vi "pirometer 2.2_MAIN.vi"() -> ()   [LabVIEW 2013]
doc: "Пирометр 2.2, разработан в ЛФВЭ ОИЯИ 2013"
uses:
  pirometer typedef1.ctl
  <vilib>/Utility/error.llb/DialogType.ctl
  <vilib>/Instr/_visa.llb/VISA Configure Serial Port (Instr).vi
  <vilib>/ptbypt/NI_PtbyPt.lvlib
panel:
  in  "Гр2":bool=TRUE
  in  "Гр1":bool=TRUE
  out "Ошибка  прибора":bool
  in  "Недопустимая \nразница между\n показаниями":u8=35
  in  "Снимок экрана":bool
  in  "Мин\n  d/dt":dbl=-0.02 min=-200.0 max=200.0 step=0.01 format="%#.3g"
  in  "Макс\n  d/dt":dbl=0.02 min=-200.0 max=200.0 step=0.01 format="%#.3g"
  out "d/dt right scale":dbl(slide) min=-0.20900000000000002 max=0.196 scale=-0.02..0.02
  out "d/dt":dynamicdata(graph)
  out "gradusnik 2":dbl(slide) scale=-3.0..35.0
  in  "Мин. Т":i8=10
  in  "Stop":bool
  out "gradusnik":dbl(slide) scale=-3.0..35.0
  in  "Усреднение d/dt":u16=25
  in  "Усреднение T по":u8=50
  out "Средняя T":dbl format="%0.2f"
  in  "Макс.Т":i8=35
  out "Температура":dynamicdata(graph)
  in  "Запись в файл":bool
  out "сек.":string="20"
  out "мин.":string="3"
  out "часы":string
  in  "xScale +":bool
  in  "Добавить время":dbl(ring)=60.0 items=["1 сек."=1.0, "10 сек."=10.0, "1 мин."=60.0, "5 мин."=300.0, "10 мин."=600.0]
  in  "xScale -":bool
  out "Текущая T":dbl format="%0.2f"
  in  "Порт":refnum<visa-resource-name>="COM7"
  out "Соединение":bool
  out "Чтение":bool
  out "Расположение файла":path=path "Запись в файл не включена..."
  in  "Бод":u32=9600
  out "d/dt":dbl format="%#.3f"
  out "Exitting":string="Остановка программы..."
  in  "index of current arr element":i32
  out "i":i32
  in  "number of data sample":u64
  out "refnum out":refnum<file>
  in  "fl_1":bool
  out "Temper.":dbl
  out "Err msg":string=" INSTRUCTIONS:\r\rNormal Use:  When using subVIs that incorporate the error in/error out (or error I/O) structure, place this handler where you want to inform the user of an error, typically at the end of the I/O data path, as the last action of the program.  If the error in error? is ERROR, the handler creates a message describing the error and its source.  If the type of dialog = 1 (default), the message is displayed to the user, who can only acknowedge it.  If the type = 2, the user can acknowledge the message or abort execution; aborting a program with active I/O is not recommended.  If the type = 0, no message is displayed; this is used to process the error programmatically, and the error out cluster elements are wired to individual terminals for that reason.  \r\rOther Use:\n\r\nlocal testing.  To test the error code of a subVI or function that does not have the error I/O structure, you can wire its error code and a source string to the local error code and error source inputs.  If error in error? indicates no error and error code is not equal to 0, the local code and source are substituted for the error in values, and error? is set TRUE (ERROR)."
  # "°С"
  # "°С"
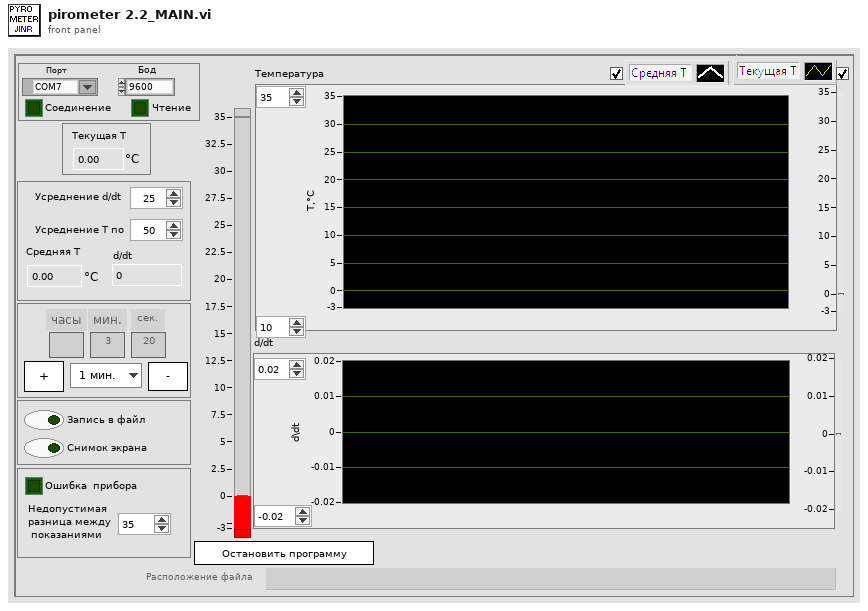
[diagram p1: front panel]
types:
  T1 = typedef "pirometer typedef1.ctl" = enum16{"Initialize", "Read port", "Averaging", "Create graph", "Save to file", "Stop", "ScreenCapture", "Err handle"}
  T2 = typedef "DialogType.ctl" = u16
  T3 = typedef "imagedata.ctl" = cluster{"image type":i32, "image depth":i32, "image":u8[], "mask":u8[], "colors":u32[], "Rectangle":cluster{"left":i16, "top":i16, "right":i16, "bottom":i16}}
  T4 = typedef "LVDateTimeRec.ctl" = cluster{"fractional second":dbl, "second":i32, "minute":i32, "hour":i32, "day of month":i32, "month":i32, "year":i32, "day of week":i32, "day of year":i32, "DST":i32}
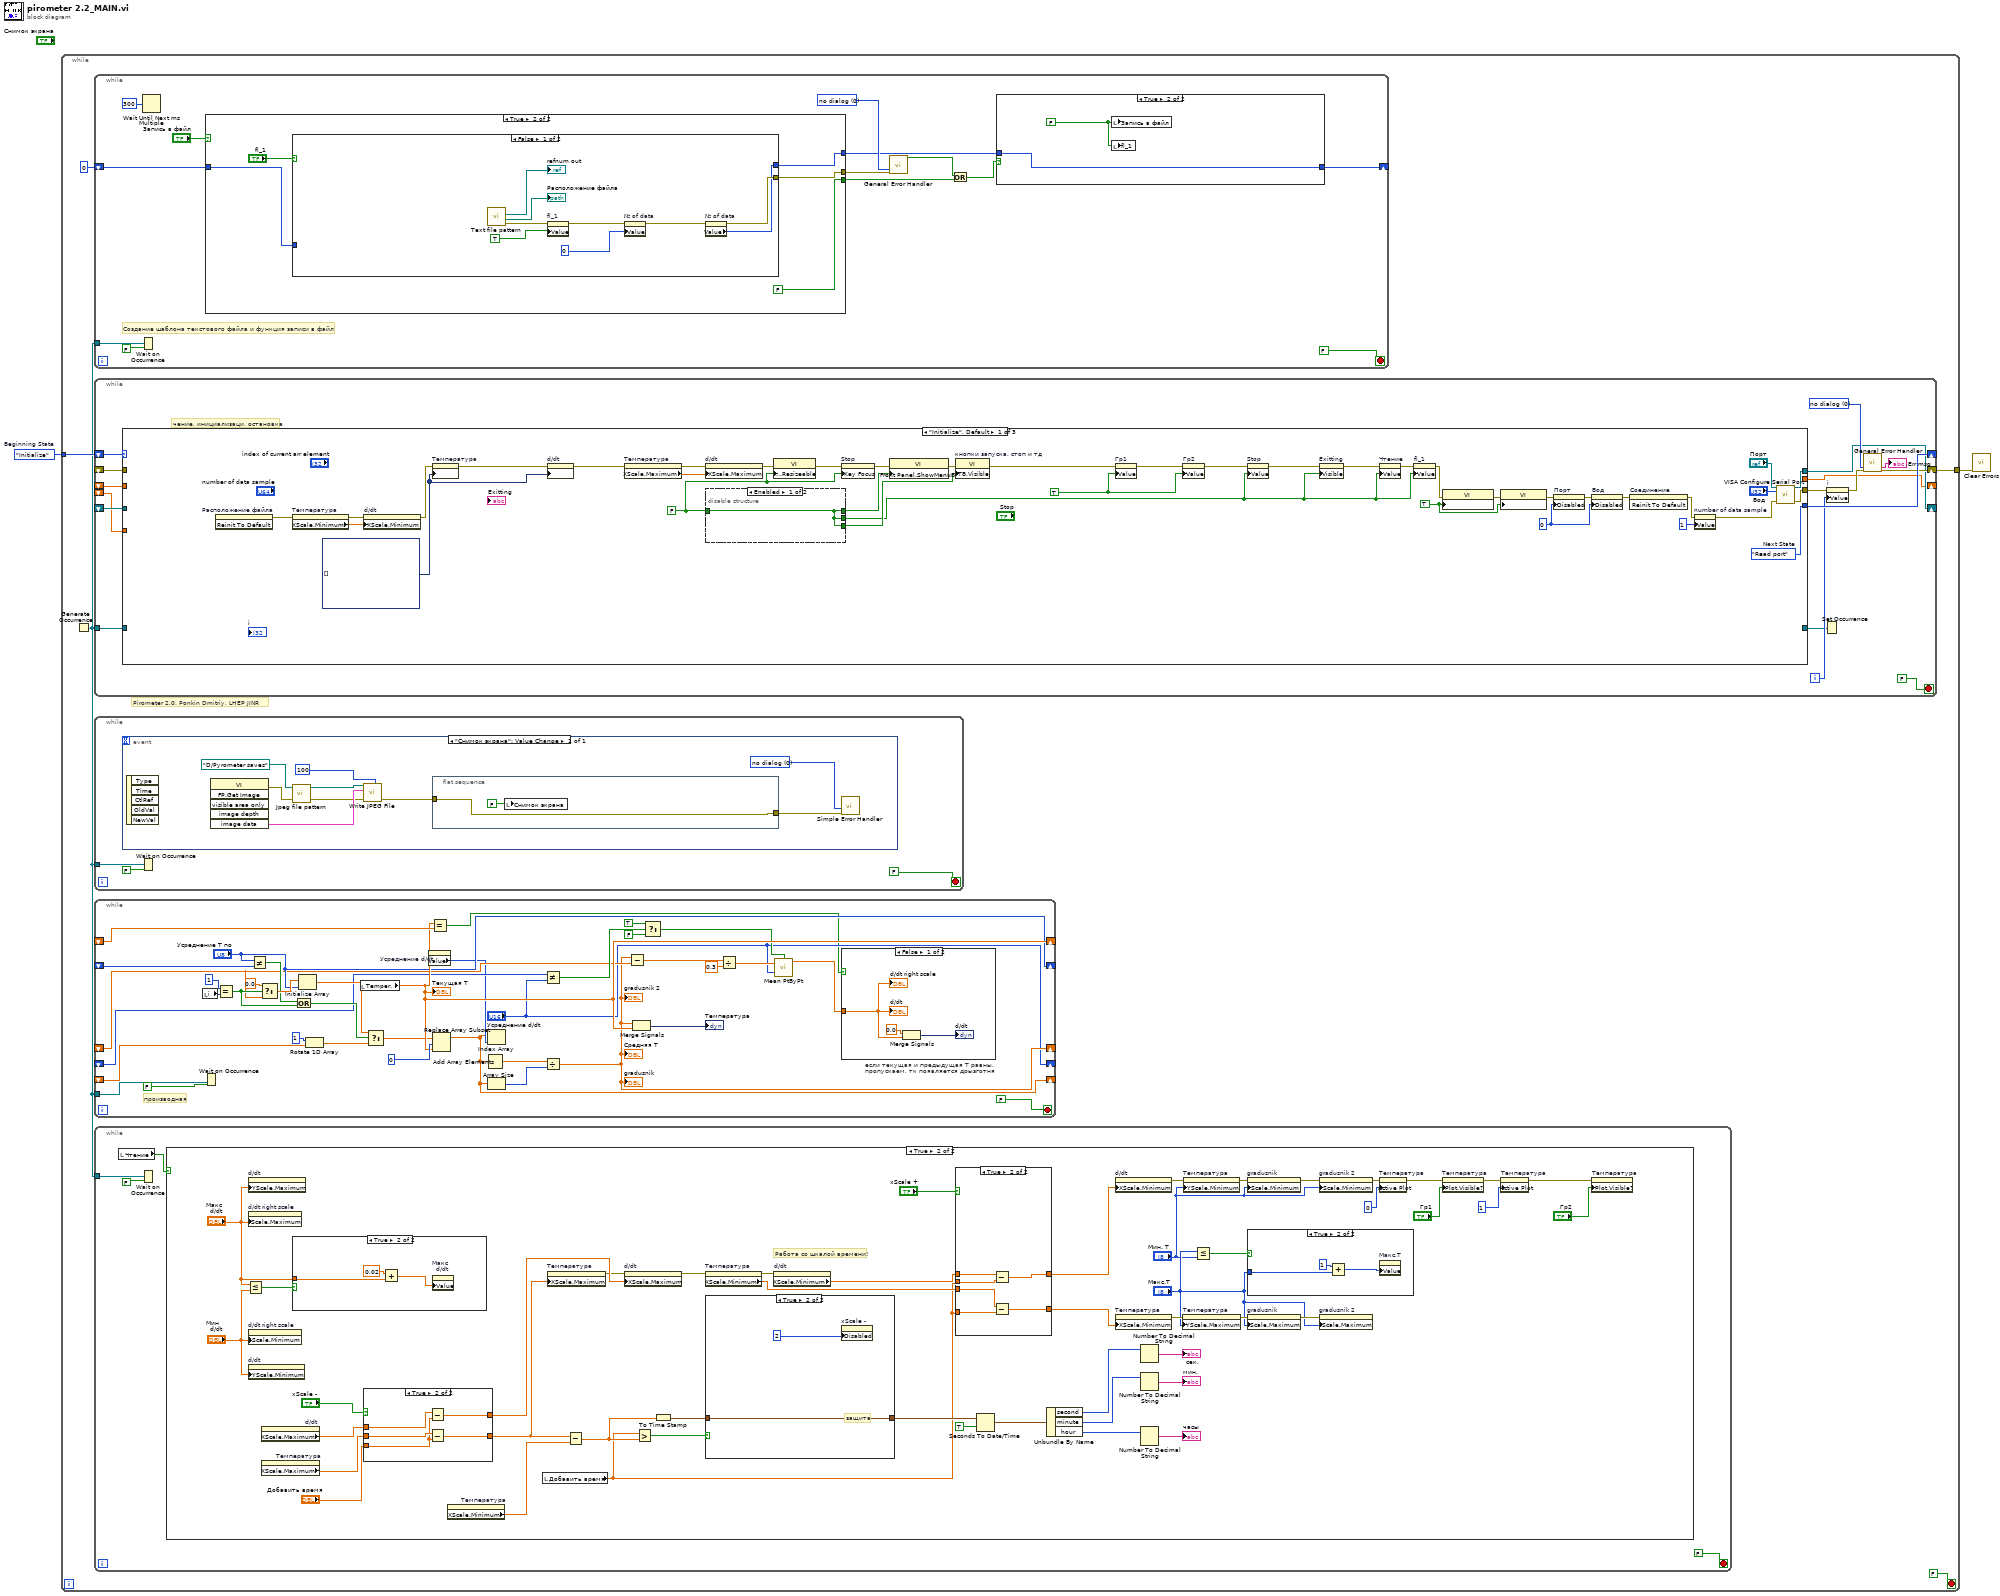
[diagram p0: block diagram]
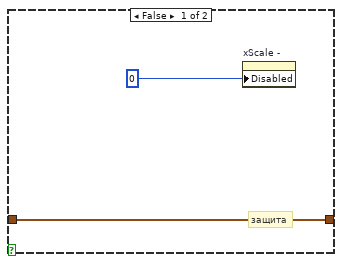
[diagram p6: hidden frame]
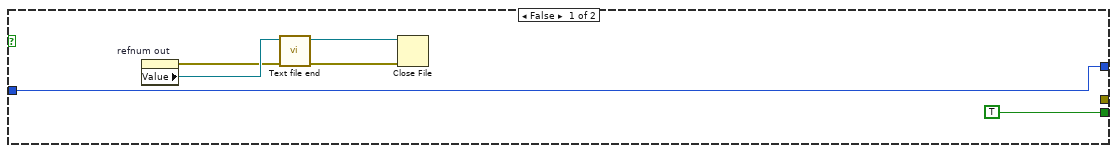
[diagram p10: hidden frame]
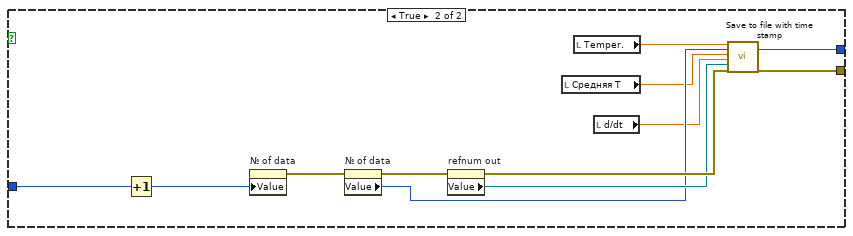
[diagram p11: hidden frame]
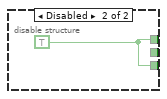
[diagram p12: hidden frame]
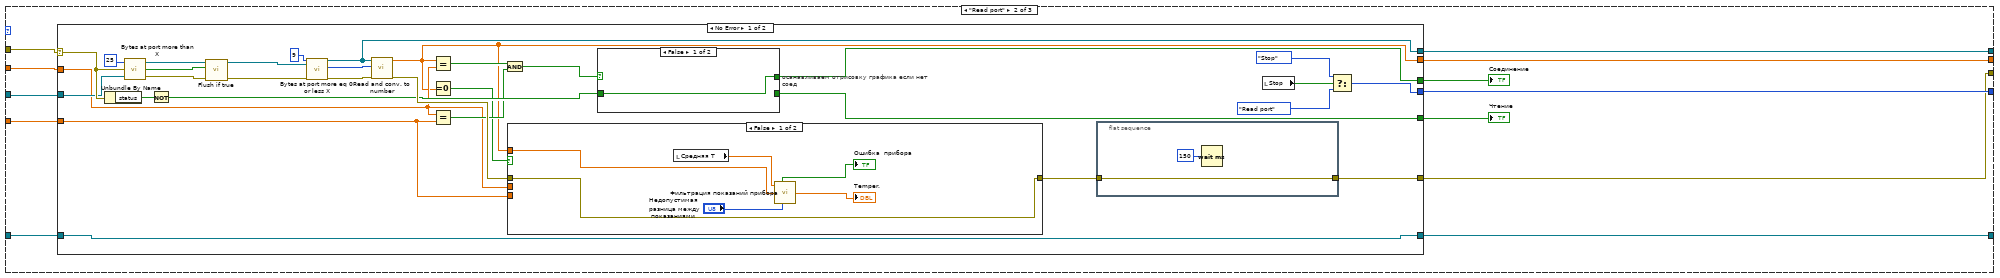
[diagram p13: hidden frame]
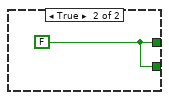
[diagram p14: hidden frame]
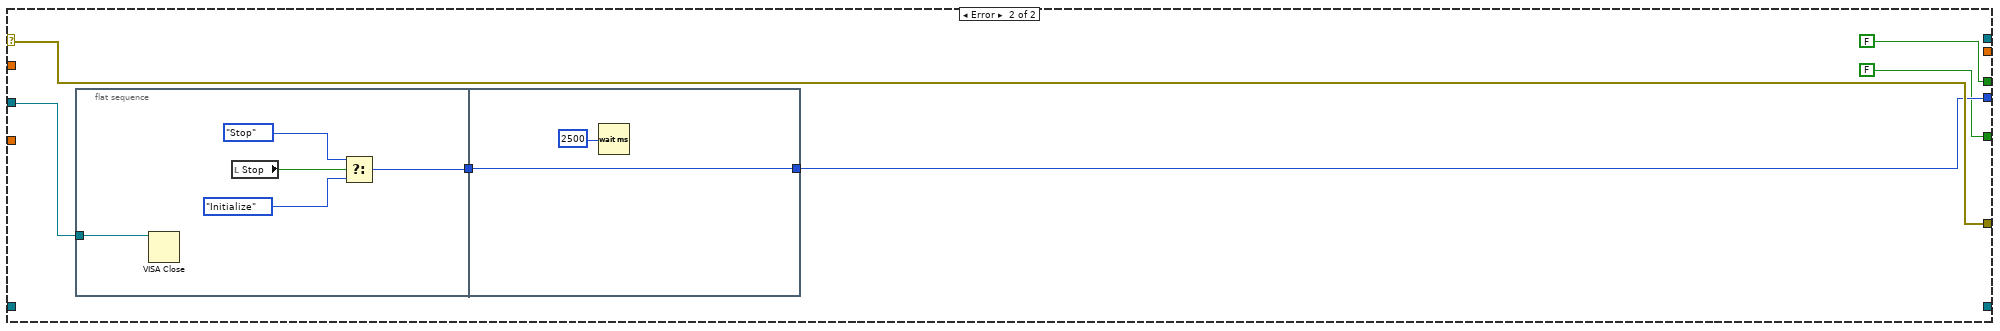
[diagram p16: hidden frame]
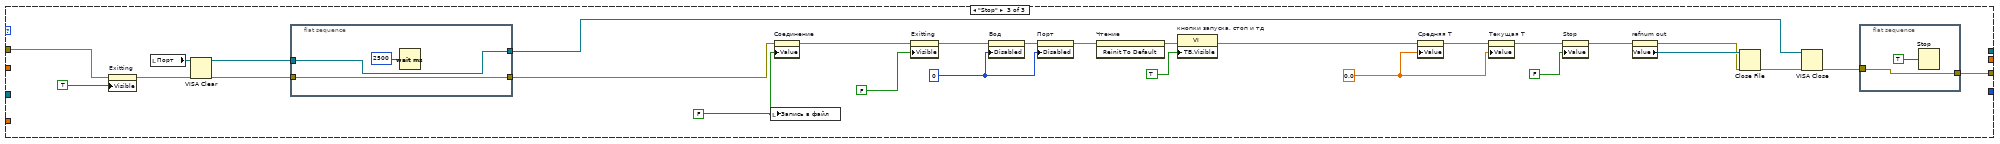
[diagram p17: hidden frame]
diagram:
  w2 = pirometer_typedef1."Initialize"  # Beginning State
  n1 = while {
    tunnel: w2 -> [w7]
    tunnel: [w5] -> w1
    stop <- FALSE stop-if-true
    # "Pirometer 2.0, Ponkin Dmitriy, LHEP JINR"
    n2 = Generate Occurrence() -> (w3:refnum<k4>)
    n3 = while {
      shift-right: [w144] -> _
      shift-left: u64 0 ("number of data sample out") -> [w152]
      tunnel: w3 -> [w151]
      stop <- FALSE stop-if-true
      w148 = T2 0 items=["no dialog", "OK message", "continue or stop message", "OK message + warnings", "continue/stop + warnings"] ("type of dialog (OK msg:1)")
      # "Создание шаблона текстового файла и функция записи в файл"
      n4 = Wait on Occurrence(1:FALSE ("ignore previous (T)"), 2:w151) -> ()  [unwired: 2 out]
      n5 = Wait Until Next ms Multiple(millisecond multiple=u32 300 ("milliseconds to wait")) -> ()  [unwired: 1 out]
      n6 = case shown="True" "Запись в файл" {
        tunnel: [_ w166] -> w146
        tunnel: [w161 w164] -> w145
        tunnel: w152 -> [w161 w163]
        tunnel: [TRUE ("save to file ?") FALSE ("save to file ?")] -> w141
        frame False {
          n7 = property on="refnum out" class="Ref (strict)"() -> (error out=w158:errorcluster, "Value"=w159:refnum<file>)  [unwired: 2 in, 1 out]
          n8 = call "Text file end.vi"("error in"=w158, "refnum file"=w159) -> ("error out"=w160:errorcluster, "refnum out"=w157:refnum<file>)  [unwired: 1 in, 7 out]
          n9 = Close File(refnum=w157, error in=w160) -> ()  [unwired: 2 out]
        }
        frame True {
          n10 = case shown="False" "fl_1" {
            tunnel: [w168 w183] -> w166
            tunnel: [w167 w179] -> w164
            tunnel: w163 -> [_ w186]
            frame False {
              n11 = call "Text file pattern.vi"() -> ("error out"=w174:errorcluster, "selected path"=→"Расположение файла":path, "refnum out"=→"refnum out":refnum<file>)  [unwired: 4 in, 5 out]
              n12 = property on="fl_1" class="Bool (strict)"(error in=w174, "Value"=TRUE ("fl_1")) -> (error out=w171:errorcluster)  [unwired: 1 in, 1 out]
              n13 = property on="№ of data" class="DigNum (strict)"(error in=w171, "Value"=u64 0 ("number of data sample")) -> (error out=w169:errorcluster)  [unwired: 1 in, 1 out]
              n14 = property on="№ of data" class="DigNum (strict)"(error in=w169) -> (error out=w168:errorcluster, "Value"=w167:u64)  [unwired: 1 in, 1 out]
            }
            frame True {
              n15 = Increment(x=w186) -> (x+1=w187:u64)
              n16 = property on="№ of data" class="DigNum (strict)"("Value"=w187) -> (error out=w184:errorcluster)  [unwired: 2 in, 1 out]
              n17 = property on="№ of data" class="DigNum (strict)"(error in=w184) -> (error out=w185:errorcluster, "Value"=w180:u64)  [unwired: 1 in, 1 out]
              n18 = property on="refnum out" class="Ref (strict)"(error in=w185) -> (error out=w182:errorcluster, "Value"=w181:refnum<file>)  [unwired: 1 in, 1 out]
              n19 = local read "Средняя T"() -> (w177:dbl)
              n20 = local read "Temper."() -> (w178:dbl)
              n21 = local read "d/dt"() -> (w176:dbl)
              n22 = call "Save to file with time stamp.vi"("T in"=w178, "number of data sample"=w180, "Average in"=w177, "d/dt in"=w176, "refnum file"=w181, "error in"=w182) -> ("number of data sample out"=w179:u64, "error out"=w183:errorcluster)  [unwired: 12 out]
            }
          }
        }
      }
      n23 = call <vilib>:"General Error Handler.vi"("type of dialog (OK msg:1)"=w148, "error in (no error)"=w146) -> ("error?"=w143:bool)  [unwired: 13 out]
      n24 = Or(x=w143, y=w141) -> (x .or. y?=w142:bool)
      n25 = case shown="True" w142 {
        tunnel: w145 -> [w153 w154]
        tunnel: [w153 w154] -> w144
        frame False {
        }
        frame True {
          w155 = FALSE ("save to file ?")
          n26 = local write "Запись в файл"(w155) -> ()
          n27 = local write "fl_1"(w155) -> ()
        }
      }
    }
    n28 = while {
      shift-right: [w203] -> _
      shift-left: w7 -> [w204]
      shift-right: [w201] -> w5
      shift-left: _ -> [w198]
      tunnel: w3 -> [w194]
      shift-right: [w193] -> _
      shift-left: _ -> [w192]
      shift-right: [w191] -> _
      shift-left: _ -> [w190]
      shift-left: _ -> [w189]
      i -> [w197]
      stop <- FALSE stop-if-true
      w200 = T2 0 items=["no dialog", "OK message", "continue or stop message", "OK message + warnings", "continue/stop + warnings"] ("type of dialog (OK msg:1)")
      # "чение, инициализаци, остановка"
      n29 = case shown="\"Initialize\", Default" w204 {
        tunnel: [w237 w257 _] -> w203
        tunnel: [w236 w253 w318] -> w196
        tunnel: w198 -> [_ w247 w340]
        tunnel: w194 -> [_ w255 _]
        tunnel: [w234 w251 _] -> w193
        tunnel: w192 -> [_ w252 _]
        tunnel: [_ w250 _] -> w191
        tunnel: w190 -> [_ w249 _]
        tunnel: w189 -> [_ w248 _]
        tunnel: [_ w246 _] -> w188
        frame "Initialize", Default {
          w235 = dynamicdata[] [] ("History Data")
          w237 = pirometer_typedef1."Read port"  # Next State
          w205 = TRUE ("Гр1")
          w228 = TRUE ("Front Panel Window:Minimizable")
          w216 = FALSE ("Front Panel Window:Resizable")
          w225 = u8 0 ("Disabled")
          n30 = invoke on="Расположение файла" class="Path" method="Reinit To Default"() -> (error out=w217:errorcluster)  [unwired: 3 in, 2 out]
          n31 = property on="Температура" class="WFChart (strict)"(error in=w217) -> (error out=w218:errorcluster, "XScale.Minimum"=w223:dbl)  [unwired: 1 in, 1 out]
          n32 = property on="d/dt" class="WFChart (strict)"(error in=w218, "XScale.Minimum"=w223) -> (error out=w219:errorcluster)  [unwired: 1 in, 1 out]
          n33 = property on="Температура" class="WFChart (strict)"(error in=w219, "History Data"=w235) -> (error out=w221:errorcluster)  [unwired: 1 in, 1 out]
          n34 = property on="d/dt" class="WFChart (strict)"(error in=w221, "History Data"=w235) -> (error out=w220:errorcluster)  [unwired: 1 in, 1 out]
          n35 = property on="Температура" class="WFChart (strict)"(error in=w220) -> (error out=w210:errorcluster, "XScale.Maximum"=w224:dbl)  [unwired: 1 in, 1 out]
          n36 = property on="d/dt" class="WFChart (strict)"(error in=w210, "XScale.Maximum"=w224) -> (error out=w222:errorcluster)  [unwired: 1 in, 1 out]
          n37 = disable-structure shown="Enabled" {
            disable-tunnel: w216 -> [w244 _]
            disable-tunnel: [w244 _] -> w212
            disable-tunnel: [w244 w245] -> w215
            disable-tunnel: [w244 w245] -> w214
            frame Enabled {
            }
            frame Disabled {
              w245 = TRUE
            }
          }
          n38 = property class="VI"(error in=w222, "Front Panel.Resizeable"=w216) -> (error out=w233:errorcluster)  [unwired: 1 in, 1 out]
          n39 = property on="Stop" class="Bool (strict)"(error in=w233, "Key Focus"=w216) -> (error out=w232:errorcluster)  [unwired: 1 in, 1 out]
          n40 = property class="VI"(error in=w232, "Front Panel.ShowMenuBar"=w215) -> (error out=w231:errorcluster)  [unwired: 1 in, 1 out]
          n41 = property on="кнопки запуска, стоп и тд" class="VI"(error in=w231, "TB.Visible"=w214) -> (error out=w206:errorcluster)  [unwired: 1 in, 1 out]
          n42 = property on="Гр1" class="Bool (strict)"(error in=w206, "Value"=w205) -> (error out=w207:errorcluster)  [unwired: 1 in, 1 out]
          n43 = property on="Гр2" class="Bool (strict)"(error in=w207, "Value"=w205) -> (error out=w208:errorcluster)  [unwired: 1 in, 1 out]
          n44 = property on="Stop" class="Bool (strict)"(error in=w208, "Value"=w212) -> (error out=w213:errorcluster)  [unwired: 1 in, 1 out]
          n45 = property on="Exitting" class="Str"(error in=w213, "Visible"=w212) -> (error out=w226:errorcluster)  [unwired: 1 in, 1 out]
          n46 = property on="Чтение" class="Bool (strict)"(error in=w226, "Value"=w212) -> (error out=w242:errorcluster)  [unwired: 1 in, 1 out]
          n47 = property on="fl_1" class="Bool (strict)"(error in=w242, "Value"=w212) -> (error out=w230:errorcluster)  [unwired: 1 in, 1 out]
          n48 = property class="VI"(error in=w230, "Front Panel.Minimizeable"=w228) -> (error out=w227:errorcluster)  [unwired: 1 in, 1 out]
          n49 = property class="VI"(error in=w227, "Front Panel.TitleBarVis"=w228) -> (error out=w209:errorcluster)  [unwired: 1 in, 1 out]
          n50 = property on="Порт" class="VISAName"(error in=w209, "Disabled"=w225) -> (error out=w211:errorcluster)  [unwired: 1 in, 1 out]
          n51 = property on="Бод" class="DigNum (strict)"(error in=w211, "Disabled"=w225) -> (error out=w238:errorcluster)  [unwired: 1 in, 1 out]
          n52 = invoke on="Соединение" class="Bool (strict)" method="Reinit To Default"(error in=w238) -> (error out=w241:errorcluster)  [unwired: 2 in, 2 out]
          n53 = property on="number of data sample" class="DigNum (strict)"(error in=w241, "Value"=u64 1 ("number of data sample")) -> (error out=w229:errorcluster)  [unwired: 1 in, 1 out]
          n54 = call-poly "VISA Configure Serial Port"("VISA resource name"="Порт", "baud rate (9600)"="Бод", "error in (no error)"=w229) -> ("VISA resource name out"=w234:refnum<visa-resource-name>, "error out"=w236:errorcluster)  [unwired: 3 in, 8 out]
        }
        frame "Read port" {
          n55 = case shown="No Error" w247 {
            selector: w247 -> [w274 w305]
            tunnel: [w271 w305] -> w253
            tunnel: [w285 w303] -> w257
            tunnel: [w267 FALSE] -> w256
            tunnel: [w266 FALSE ("Reading data")] -> w254
            tunnel: [w277 _] -> w246
            tunnel: w255 -> [w277 _]
            tunnel: w252 -> [w270 w300]
            tunnel: [w269 _] -> w251
            tunnel: [w260 _] -> w250
            tunnel: w249 -> [w262 _]
            tunnel: w248 -> [w261 _]
            frame No Error {
              n56 = Unbundle By Name(w274) -> ("status"=w273:bool)
              n57 = call "Bytes at port more than X.vi"("X"=u32 25, "error IO"=w274, "port in"=w270) -> ("port out"=w282:refnum<visa-resource-name>, "Bytes at port > X"=w283:bool, "error out"=w284:errorcluster)  [unwired: 4 out]
              n58 = Not(x=w273) -> (.not. x?=w268:bool)
              n59 = call "Flush if true.vi"("error in"=w284, "Bytes at port > X"=w283, "port in"=w282) -> ("error out"=w281:errorcluster, "port out"=w280:refnum<visa-resource-name>)  [unwired: 7 out]
              n60 = call "Bytes at port more eq 0 or less X.vi"("X"=u32 9, "serial ref  name"=w280, "error IO"=w281) -> ("serial out"=w269:refnum<visa-resource-name>, "Num. of Bytes at Port"=w278:u32, "error out"=w279:errorcluster)  [unwired: 2 in, 12 out]
              n61 = call "Read and conv. to number.vi"("error in"=w279, "Num. of Bytes at Port"=w278, "port"=w269) -> ("error out"=w276:errorcluster, "Temper."=w260:dbl)  [unwired: 1 in, 6 out]
              n62 = Equal?(x=w260, y=w262) -> (x = y?=w264:bool)
              n63 = Equal To 0?(x=w260) -> (x = 0?=w259:bool)
              n64 = Equal?(x=w262, y=w261) -> (x = y?=w263:bool)
              n65 = And(x=w264, y=w263) -> (x .and. y?=w265:bool)
              n66 = case shown="False" w259 {
                tunnel: w276 -> [w298 w299]
                tunnel: [w298 w299] -> w272
                tunnel: w260 -> [w294 _]
                tunnel: w262 -> [_ _]
                tunnel: w261 -> [_ _]
                frame False {
                  n67 = local read "Средняя T"() -> (w293:dbl)
                  n68 = call "Фильтрация показаний прибора.vi"("Среднее"=w293, "Текущее показание"=w294, "Разница между \nпоказаниями прибора"="Недопустимая \nразница между\n показаниями") -> ("Ошибка \nприбора"=→"Ошибка  прибора":bool, "Отфильтрован.\nвеличина"=→"Temper.":dbl)  [unwired: 1 in, 4 out]
                }
                frame True {
                }
              }
              n69 = case "осанавливаем отрисовку графика если нет соед" shown="False" w265 {
                tunnel: w268 -> [w289 _]
                tunnel: [w289 w290] -> w267
                tunnel: [_ w290] -> w266
                frame False {
                }
                frame True {
                  w290 = FALSE
                }
              }
              n70 = flat-sequence {
                tunnel: w272 -> [w292]
                tunnel: [w292] -> w271
                frame #0 {
                  n71 = Wait (ms)(milliseconds to wait=u32 150) -> ()  [unwired: 1 out]
                }
              }
              n72 = local read "Stop"() -> (w275:bool)
              n73 = Select(t=pirometer_typedef1."Stop" ("Beginning State"), s=w275, f=pirometer_typedef1."Read port" ("Beginning State")) -> (s? t:f=w285:T1)
            }
            frame Error {
              n74 = flat-sequence {
                tunnel: [w307] -> w304
                tunnel: w300 -> [w306]
                tunnel: [w311] -> w303
                tunnel: w304 -> [w311]
                frame #0 {
                  n75 = VISA Close(VISA resource name=w306) -> ()  [unwired: 1 in, 1 out]
                  n76 = local read "Stop"() -> (w310:bool)
                  n77 = Select(t=pirometer_typedef1."Stop" ("Beginning State"), s=w310, f=pirometer_typedef1."Initialize" ("Beginning State")) -> (s? t:f=w307:T1)
                }
                frame #1 {
                  n78 = Wait (ms)(milliseconds to wait=u32 2500) -> ()  [unwired: 1 out]
                }
              }
            }
          }
          "Соединение" <- w256
          "Чтение" <- w254
        }
        frame "Stop" {
          w324 = 0.0 ("Текущая T")
          w314 = u8 0 ("Disabled")
          w336 = FALSE ("Connected")
          n79 = property on="Exitting" class="Str"(error in=w340, "Visible"=TRUE) -> (error out=w337:errorcluster)  [unwired: 1 in, 1 out]
          n80 = local read "Порт"() -> (w339:refnum<visa-resource-name>)
          n81 = VISA Clear(VISA resource name=w339, error in (no error)=w337) -> (VISA resource name out=w322:refnum<visa-resource-name>, error out=w320:errorcluster)
          n82 = flat-sequence {
            tunnel: w322 -> [w342]
            tunnel: [w342] -> w321
            tunnel: [w341] -> w319
            tunnel: w320 -> [w341]
            frame #0 {
              n83 = Wait (ms)(milliseconds to wait=u32 2500) -> ()  [unwired: 1 out]
            }
          }
          n84 = local write "Запись в файл"(w336) -> ()
          n85 = property on="Соединение" class="Bool (strict)"(error in=w319, "Value"=w336) -> (error out=w315:errorcluster)  [unwired: 1 in, 1 out]
          n86 = property on="Exitting" class="Str"(error in=w315, "Visible"=FALSE) -> (error out=w313:errorcluster)  [unwired: 1 in, 1 out]
          n87 = property on="Бод" class="DigNum (strict)"(error in=w313, "Disabled"=w314) -> (error out=w333:errorcluster)  [unwired: 1 in, 1 out]
          n88 = property on="Порт" class="VISAName"(error in=w333, "Disabled"=w314) -> (error out=w332:errorcluster)  [unwired: 1 in, 1 out]
          n89 = invoke on="Чтение" class="Bool (strict)" method="Reinit To Default"(error in=w332) -> (error out=w334:errorcluster)  [unwired: 2 in, 2 out]
          n90 = property on="кнопки запуска, стоп и тд" class="VI"(error in=w334, "TB.Visible"=TRUE ("Tool Bar:Visible")) -> (error out=w326:errorcluster)  [unwired: 1 in, 1 out]
          n91 = property on="Средняя T" class="DigNum (strict)"(error in=w326, "Value"=w324) -> (error out=w325:errorcluster)  [unwired: 1 in, 1 out]
          n92 = property on="Текущая T" class="DigNum (strict)"(error in=w325, "Value"=w324) -> (error out=w327:errorcluster)  [unwired: 1 in, 1 out]
          n93 = property on="Stop" class="Bool (strict)"(error in=w327, "Value"=FALSE ("Stop")) -> (error out=w329:errorcluster)  [unwired: 1 in, 1 out]
          n94 = property on="refnum out" class="Ref (strict)"(error in=w329) -> (error out=w330:errorcluster, "Value"=w331:refnum<file>)  [unwired: 1 in, 1 out]
          n95 = Close File(refnum=w331, error in=w330) -> (error out=w316:errorcluster)  [unwired: 1 out]
          n96 = VISA Close(VISA resource name=w321, error in (no error)=w316) -> (error out=w317:errorcluster)
          n97 = flat-sequence {
            tunnel: [w345] -> w318
            tunnel: w317 -> [w345]
            frame #0 {
              n98 = Stop(stop? (T)=TRUE) -> ()
            }
          }
        }
      }
      n99 = Set Occurrence(w188) -> ()
      n100 = property on="i" class="DigNum (strict)"(error in=w196, "Value"=w197) -> (error out=w195:errorcluster)  [unwired: 1 in, 1 out]
      n101 = call <vilib>:"General Error Handler.vi"("type of dialog (OK msg:1)"=w200, "error in (no error)"=w195) -> ("message"=→"Err msg":string, "error out"=w201:errorcluster)  [unwired: 12 out]
    }
    n102 = while {
      tunnel: w3 -> [w8]
      stop <- FALSE stop-if-true
      n103 = event shown="[0] \"Снимок экрана\": Value Change" {
        selector: _ -> [_]
        dyn-events: _ -> [_]
        timeout: _ -> [_]
        event "Снимок экрана": Value Change {
          w12 = T2 0 items=["no dialog", "OK message", "continue or stop message", "OK message + warnings", "continue/stop + warnings"] ("type of dialog (OK msg:1)")
          n104 = event-data() -> ()  [unwired: 6 out]
          n105 = invoke class="VI" method="FP.Get Image"() -> (error out=w17:errorcluster, "image data"=w18:T3)  [unwired: 6 in, 4 out]
          n106 = call "Jpeg file pattern.vi"("path"=path "D:/Pyrometer saves", "error in"=w17) -> ("path to JPG file"=w16:path, "error out"=w15:errorcluster)  [unwired: 6 out]
          n107 = call <vilib>:"Write JPEG File.vi"("quality (80)"=100, "error in (no error)"=w15, "image data"=w18, "path to JPEG file"=w16) -> ("error out"=w13:errorcluster)  [unwired: 7 out]
          n108 = flat-sequence {
            tunnel: w13 -> [w20]
            tunnel: [w20] -> w11
            frame #0 {
              n109 = local write "Снимок экрана"(FALSE ("Снимок экрана")) -> ()
            }
          }
          n110 = call <vilib>:"Simple Error Handler.vi"("type of dialog (OK msg:1)"=w12, "error in (no error)"=w11) -> ()  [unwired: 8 out]
        }
      }
      n111 = Wait on Occurrence(1:FALSE ("ignore previous (T)"), 2:w8) -> ()  [unwired: 1 in, 1 out]
    }
    n112 = while {
      shift-right: [w24] -> _
      shift-left: _ -> [w59]
      tunnel: w3 -> [w56]
      shift-right: ["Усреднение T по"] -> _
      shift-left: _ -> [w55]
      shift-right: [w30] -> _
      shift-left: _ -> [w31]
      shift-right: [w40] -> _
      shift-left: _ -> [w41]
      shift-right: ["Усреднение d/dt"] -> _
      shift-left: _ -> [w33]
      stop <- FALSE stop-if-true
      # "производная"
      n113 = local read "i"() -> (w27:i32)
      n114 = Wait on Occurrence(1:FALSE ("ignore previous (T)"), 2:w56) -> ()  [unwired: 1 in, 1 out]
      n115 = Equal?(x=1 ("y"), y=w27) -> (x = y?=w53:bool)
      n116 = Not Equal?(x="Усреднение T по", y=w55) -> (x != y?=w50:bool)
      n117 = Select(t=0.0, s=w53, f=w31) -> (s? t:f=w51:dbl)
      n118 = Or(x=w50, y=w53) -> (x .or. y?=w49:bool)
      n119 = Initialize Array(w51, "Усреднение T по") -> (w44:dbl[])
      n120 = Rotate 1D Array(1:w59, 2:1 ("n")) -> (0:w46:dbl[])
      n121 = local read "Temper."() -> (w40:dbl)
      "Текущая T" <- w40
      n122 = Select(t=w44, s=w49, f=w46) -> (s? t:f=w26:dbl[])
      n123 = property on="Усреднение d/dt" class="DigNum (strict)"() -> ("Value"=w25:u16)  [unwired: 2 in, 2 out]
      n124 = Equal?(x=w40, y=w41) -> (x = y?=w22:bool)
      n125 = Replace Array Subset(array=w26, new element=w40, index=0) -> (w24:dbl[])
      n126 = Add Array Elements(numeric array=w24) -> (sum=w54:dbl)
      n127 = Index Array(array=w24, index=w25) -> ()  [unwired: 1 out]
      n128 = Array Size(array=w24) -> (size(s)=w29:i32)
      n129 = Not Equal?(x=w33, y="Усреднение d/dt") -> (x != y?=w34:bool)
      n130 = Divide(x=w54, y=w29) -> (x/y=w30:dbl)
      "Средняя T" <- w30
      "gradusnik" <- w30
      "gradusnik 2" <- w30
      n131 = Subtract(x=w30, y=w31) -> (x-y=w43:dbl)
      n132 = Merge Signals(w30, w40) -> (→"Температура":dynamicdata)
      n133 = Select(t=TRUE ("initialize"), s=w34, f=FALSE ("initialize")) -> (s? t:f=w32:bool)
      n134 = Divide(x=w43, y=0.3 ("dT")) -> (x/y=w37:dbl)
      n135 = call <vilib>:"Mean PtByPt.vi"("x"=w37, "sample length"="Усреднение d/dt", "initialize"=w32) -> ("mean"=w38:dbl)  [unwired: 2 out]
      n136 = case "если текущая и предыдущая Т равны, пропускаем, тк появляется дрызготня" shown="False" w22 {
        tunnel: w38 -> [w60 _]
        frame False {
          n137 = Merge Signals(0.0 ("f"), w60) -> (→"d/dt":dynamicdata)
          "d/dt" <- w60
          "d/dt right scale" <- w60
        }
        frame True {
        }
      }
    }
    n138 = while {
      tunnel: w3 -> [w63]
      stop <- FALSE stop-if-true
      n139 = local read "Чтение"() -> (w65:bool)
      n140 = Wait on Occurrence(1:FALSE ("ignore previous (T)"), 2:w63) -> ()  [unwired: 1 in, 1 out]
      n141 = case shown="True" w65 {
        frame False {
        }
        frame True {
          # "Работа со шкалой времени!"
          n142 = Less Or Equal?(x="Макс\n  d/dt", y="Мин\n  d/dt") -> (x <= y?=w83:bool)
          n143 = property on="d/dt" class="WFChart (strict)"("YScale.Maximum"="Макс\n  d/dt") -> ()  [unwired: 2 in, 2 out]
          n144 = property on="d/dt right scale" class="Slide (strict)"("Scale.Maximum"="Макс\n  d/dt") -> ()  [unwired: 2 in, 2 out]
          n145 = property on="d/dt right scale" class="Slide (strict)"("Scale.Minimum"="Мин\n  d/dt") -> ()  [unwired: 2 in, 2 out]
          n146 = property on="d/dt" class="WFChart (strict)"("YScale.Minimum"="Мин\n  d/dt") -> ()  [unwired: 2 in, 2 out]
          n147 = property on="d/dt" class="WFChart (strict)"() -> ("XScale.Maximum"=w95:dbl)  [unwired: 2 in, 2 out]
          n148 = property on="Температура" class="WFChart (strict)"() -> ("XScale.Maximum"=w103:dbl)  [unwired: 2 in, 2 out]
          n149 = case shown="True" w83 {
            tunnel: "Макс\n  d/dt" -> [_ w120]
            frame False {
            }
            frame True {
              n150 = Add(x=0.02, y=w120) -> (x+y=w118:dbl)
              n151 = property on="Макс\n  d/dt" class="DigNum (strict)"("Value"=w118) -> ()  [unwired: 2 in, 2 out]
            }
          }
          n152 = case shown="True" "xScale -" {
            tunnel: w103 -> [w126 w130]
            tunnel: [w126 w131] -> w96
            tunnel: "Добавить время" -> [_ w128]
            tunnel: w95 -> [w125 w129]
            tunnel: [w125 w127] -> w94
            frame False {
            }
            frame True {
              n153 = Subtract(x=w129, y=w128) -> (x-y=w127:dbl)
              n154 = Subtract(x=w130, y=w128) -> (x-y=w131:dbl)
            }
          }
          n155 = property on="Температура" class="WFChart (strict)"() -> ("XScale.Minimum"=w101:dbl)  [unwired: 2 in, 2 out]
          n156 = local read "Добавить время"() -> (w75:dbl)
          n157 = property on="Температура" class="WFChart (strict)"("XScale.Maximum"=w96) -> (error out=w91:errorcluster)  [unwired: 2 in, 1 out]
          n158 = Subtract(x=w96, y=w101) -> (x-y=w106:dbl)
          n159 = property on="d/dt" class="WFChart (strict)"(error in=w91, "XScale.Maximum"=w94) -> (error out=w90:errorcluster)  [unwired: 1 in, 1 out]
          n160 = Greater?(x=w75, y=w106) -> (0:w105:bool)
          n161 = To Time Stamp(1:w106) -> (0:w99:timestamp)
          n162 = property on="Температура" class="WFChart (strict)"(error in=w90) -> (error out=w88:errorcluster, "XScale.Minimum"=w89:dbl)  [unwired: 1 in, 1 out]
          n163 = case shown="True" w105 {
            tunnel: [w121 w123] -> w98
            tunnel: w99 -> [w121 w123]
            frame False {
              # "защита"
              n164 = property on="xScale -" class="Bool"("Disabled"=u8 0) -> ()  [unwired: 2 in, 2 out]
            }
            frame True {
              # "защита"
              n165 = property on="xScale -" class="Bool"("Disabled"=u8 2) -> ()  [unwired: 2 in, 2 out]
            }
          }
          n166 = property on="d/dt" class="WFChart (strict)"(error in=w88) -> ("XScale.Minimum"=w93:dbl)  [unwired: 1 in, 2 out]
          n167 = case shown="True" "xScale +" {
            tunnel: w89 -> [w133 w139]
            tunnel: [w133 w138] -> w97
            tunnel: w75 -> [_ w137]
            tunnel: w93 -> [w132 w136]
            tunnel: w75 -> [_ w135]
            tunnel: [w132 w134] -> w92
            frame False {
            }
            frame True {
              n168 = Subtract(x=w136, y=w135) -> (x-y=w134:dbl)
              n169 = Subtract(x=w139, y=w137) -> (x-y=w138:dbl)
            }
          }
          n170 = Seconds To Date/Time(time stamp (now)=w98, to UTC (F)=TRUE) -> (date time rec=w108:T4)
          n171 = Unbundle By Name(w108) -> ("second"=w109:i32, "minute"=w110:i32, "hour"=w111:i32)
          n172 = property on="d/dt" class="WFChart (strict)"("XScale.Minimum"=w92) -> (error out=w86:errorcluster)  [unwired: 2 in, 1 out]
          n173 = property on="Температура" class="WFChart (strict)"("XScale.Minimum"=w97) -> (error out=w87:errorcluster)  [unwired: 2 in, 1 out]
          n174 = Number To Decimal String(number=w109) -> (decimal integer string=→"сек.":string)  [unwired: 1 out]
          n175 = Number To Decimal String(number=w110) -> (decimal integer string=→"мин.":string)  [unwired: 1 out]
          n176 = Number To Decimal String(number=w111) -> (decimal integer string=→"часы":string)  [unwired: 1 out]
          n177 = property on="Температура" class="WFChart (strict)"(error in=w87, "YScale.Maximum"="Макс.Т") -> (error out=w85:errorcluster)  [unwired: 1 in, 1 out]
          n178 = property on="Температура" class="WFChart (strict)"(error in=w86, "YScale.Minimum"="Мин. Т") -> (error out=w84:errorcluster)  [unwired: 1 in, 1 out]
          n179 = Less Or Equal?(x="Макс.Т", y="Мин. Т") -> (x <= y?=w78:bool)
          n180 = property on="gradusnik" class="Slide (strict)"(error in=w84, "Scale.Minimum"="Мин. Т") -> (error out=w81:errorcluster)  [unwired: 1 in, 1 out]
          n181 = case shown="True" w78 {
            tunnel: "Макс.Т" -> [_ w117]
            frame False {
            }
            frame True {
              n182 = Add(x=i8 1, y=w117) -> (x+y=w115:i8)
              n183 = property on="Макс.Т" class="DigNum (strict)"("Value"=w115) -> ()  [unwired: 2 in, 2 out]
            }
          }
          n184 = property on="gradusnik" class="Slide (strict)"(error in=w85, "Scale.Maximum"="Макс.Т") -> (error out=w82:errorcluster)  [unwired: 1 in, 1 out]
          n185 = property on="gradusnik 2" class="Slide (strict)"(error in=w81, "Scale.Minimum"="Мин. Т") -> (error out=w67:errorcluster)  [unwired: 1 in, 1 out]
          n186 = property on="gradusnik 2" class="Slide (strict)"(error in=w82, "Scale.Maximum"="Макс.Т") -> ()  [unwired: 1 in, 2 out]
          n187 = property on="Температура" class="WFChart (strict)"(error in=w67, "Active Plot"=u32 0) -> (error out=w72:errorcluster)  [unwired: 1 in, 1 out]
          n188 = property on="Температура" class="WFChart (strict)"(error in=w72, "Plot.Visible?"="Гр1") -> (error out=w71:errorcluster)  [unwired: 1 in, 1 out]
          n189 = property on="Температура" class="WFChart (strict)"(error in=w71, "Active Plot"=u32 1) -> (error out=w70:errorcluster)  [unwired: 1 in, 1 out]
          n190 = property on="Температура" class="WFChart (strict)"(error in=w70, "Plot.Visible?"="Гр2") -> ()  [unwired: 1 in, 2 out]
        }
      }
    }
  }
  n191 = call <vilib>:"Clear Errors.vi"("error in (no error)"=w1) -> ()  [unwired: 7 out]
